vi "Horn Control Loop.vi"(8 "error in (no error)":errorcluster) -> ()   [LabVIEW 2011]
uses:
  Apendage State.ctl
  <vilib>/Rock Robotics/WPI/Solenoid/WPI_SolenoidValue.ctl
  Robot Global Data.vi
  <vilib>/Rock Robotics/WPI/Solenoid/WPI_SolenoidSetEnum.vi
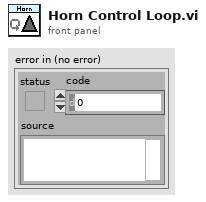
[diagram p1: front panel]
types:
  T1 = typedef "WPI_SolenoidValue.ctl" = enum16{"Off", "On", "Forward", "Reverse"}
  T2 = typedef "Apendage State.ctl" = enum16{"Unknown", "Down", "Up"}
  T3 = typedef "WPI_SolenoidDevRef.ctl" = cluster{"DevStatus":errorcluster, "Solenoid Module":T4, "Forward Solenoid Channel":T5, "Reverse Solenoid Channel":T5}
  T4 = typedef "FPGA_TypedefSolenoidModule.ctl" = enum16{"Solenoid Module 1", "Solenoid Module 2"}
  T5 = typedef "WPI_SolenoidChannel.ctl" = enum8{"Solenoid 1", "Solenoid 2", "Solenoid 3", "Solenoid 4", "Solenoid 5", "Solenoid 6", "Solenoid 7", "Solenoid 8", "Invalid"}
  T6 = typedef "WPI_RelayDevRef.ctl" = cluster{"DevStatus":errorcluster, "Relay Channel":T7, "Digital Module":T8, "Relay Direction":T9}
  T7 = typedef "FPGA_DIORelayChannel.ctl" = enum8{"Relay 1", "Relay 2", "Relay 3", "Relay 4", "Relay 5", "Relay 6", "Relay 7", "Relay 8", "Invalid"}
  T8 = typedef "FPGA_TypedefDigitalModule.ctl" = enum16{"Digital Module 1", "Digital Module 2"}
  T9 = typedef "WPI_RelayDirection.ctl" = enum16{"Both directions", "Forward only", "Reverse only"}
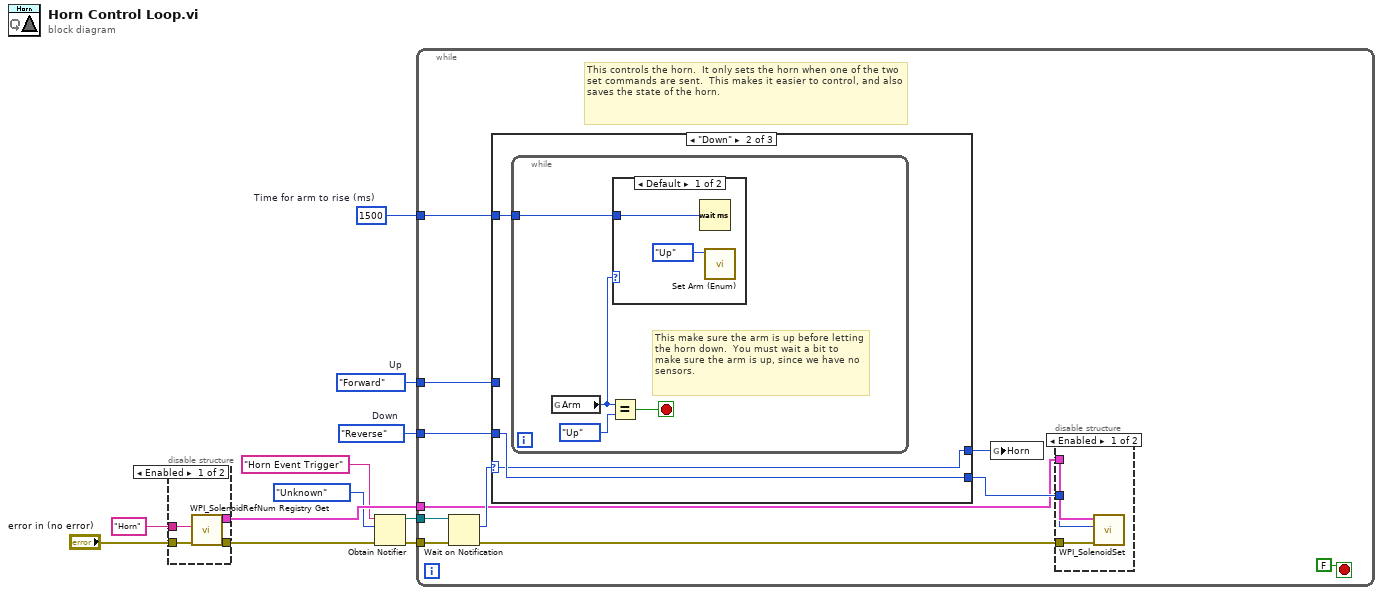
[diagram p0: block diagram]
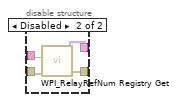
[diagram p2: hidden frame]
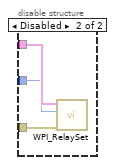
[diagram p3: hidden frame]
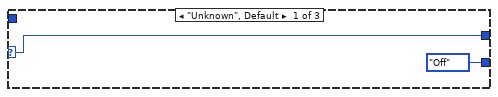
[diagram p4: hidden frame]
diagram:
  w1 = u32 1500  # Time for arm to rise (ms)
  w2 = WPI_SolenoidValue."Forward"  # Up
  w3 = WPI_SolenoidValue."Reverse"  # Down
  n1 = disable-structure shown="Enabled" {
    disable-tunnel: [w15 w16] -> w9
    disable-tunnel: [w14 w19] -> w8
    disable-tunnel: "error in (no error)" -> [w13 w18]
    disable-tunnel: "Horn" ("refnum name") -> [w12 w17]
    frame Enabled {
      n2 = call <vilib>:"WPI_SolenoidRefNum Registry Get.vi"("error in (no error)"=w13, "refnum name"=w12) -> ("error out"=w14:errorcluster, "SolenoidDevRef"=w15:T3)  [unwired: 8 in]
    }
    frame Disabled {
      n3 = call <vilib>:"WPI_RelayRefNum Registry Get.vi"("error in (no error)"=w18, "refnum name"=w17) -> ("error out"=w19:errorcluster, "RelayDevRef"=w16:T6)  [unwired: 8 in]
    }
  }
  n4 = Obtain Notifier(name (unnamed)="Horn Event Trigger", notification data type=Apendage_State."Unknown", error in (no error)=w8) -> (notifier out=w11:refnum<notifier>, error out=w10:errorcluster)  [unwired: 1 in, 1 out]
  n5 = while {
    tunnel: w11 -> [w30]
    tunnel: w10 -> [w29]
    tunnel: w9 -> [w20]
    tunnel: w3 -> [w26]
    tunnel: w2 -> [w25]
    tunnel: w1 -> [w23]
    stop <- FALSE stop-if-true
    # "This controls the horn.  It only sets the horn when one of the two set commands are sent.  This makes it easier to control, and also saves the state of the horn."
    n6 = Wait on Notification(notifier=w30, error in (no error)=w29) -> (notification=w27:T2, error out=w22:errorcluster)  [unwired: 2 in, 2 out]
    n7 = case shown="\"Down\"" w27 {
      selector: w27 -> [w37 w40 w48]
      tunnel: [WPI_SolenoidValue."Off" ("t") w41 w49] -> w21
      tunnel: w26 -> [_ w41 _]
      tunnel: w25 -> [_ _ w49]
      tunnel: [w37 w40 w48] -> w24
      tunnel: w23 -> [_ w39 _]
      frame "Unknown", Default {
      }
      frame "Down" {
        n8 = while {
          tunnel: w39 -> [w42]
          stop <- w45 stop-if-true
          # "This make sure the arm is up before letting the horn down.  You must wait a bit to make sure the arm is up, since we have no sensors."
          n9 = global read "Robot Global Data.vi" "Arm"() -> (w43:T2)
          n10 = Equal?(x=w43, y=Apendage_State."Up" ("x")) -> (x = y?=w45:bool)
          n11 = case shown="Default" w43 {
            tunnel: w42 -> [w46 _]
            frame Default {
              n12 = Wait (ms)(milliseconds to wait=w46) -> ()  [unwired: 1 out]
              n13 = call "Set Arm (Enum).vi"("Arm"=enum16{"Down", "Up"}."Up") -> ()  [unwired: 10 in, 1 out]
            }
            frame "Up" {
            }
          }
        }
      }
      frame "Up" {
      }
    }
    n14 = global write "Robot Global Data.vi" "Horn"(w24) -> ()
    n15 = disable-structure shown="Enabled" {
      disable-tunnel: w22 -> [w33 w35]
      disable-tunnel: w20 -> [w32 w36]
      disable-tunnel: w21 -> [w31 w34]
      frame Enabled {
        n16 = call-poly <vilib>:"WPI_SolenoidSet.vi"("error in (no error)"=w33, "Value"=w31, "SolenoidDevRef"=w32) -> ()  [unwired: 7 in, 2 out]
      }
      frame Disabled {
        n17 = call <vilib>:"WPI_RelaySet.vi"("error in (no error)"=w35, "RelayValue"=w34, "RelayDevRef"=w36) -> ()  [unwired: 7 in, 2 out]
      }
    }
  }
